vi "Decode Publish Package.vi"(8 "error in (no error)":errorcluster, 10 "PUBLISH in":refnum<class "PUBLISH.lvclass">, 11 "Server in":refnum<class "Server.lvclass">) -> (0 "error out":errorcluster, 1 "Payload":variant, 2 "Topic":string, 3 "Server out":refnum<class "Server.lvclass">)   [LabVIEW 2013, in "MQTT Server.lvlib" / "Server.lvclass"]
uses:
  Server.lvclass
  Control Packets/PUBLISH/PUBLISH.lvclass
  <vilib>/LabVIEW Open Source Project/Configuration Manager/Serializer/Serializer.lvclass
  Control Packets/ControlPacket/ControlPacket.lvclass/ControlPacket.ctl
  Control Packets/ControlPacket/ControlPacket.lvclass
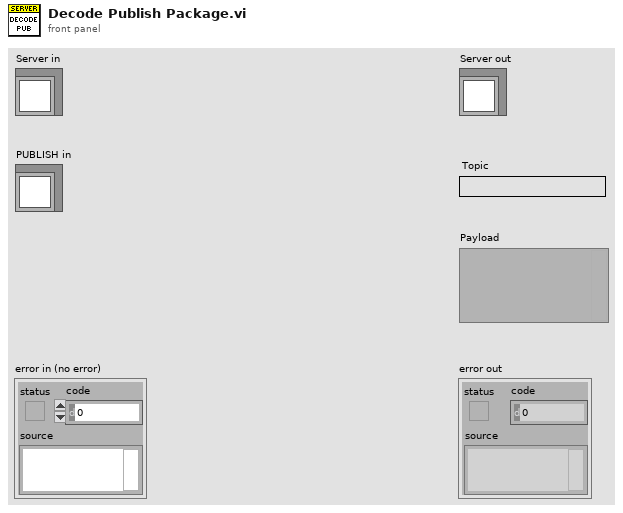
[diagram p1: front panel]
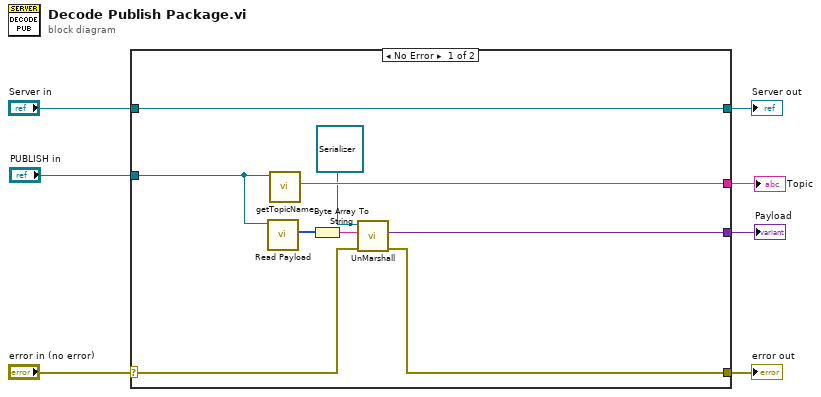
[diagram p0: block diagram]
diagram:
  n1 = case shown="No Error" "error in (no error)" {
    selector: "error in (no error)" -> [w9 w18]
    tunnel: [w8 w18] -> w6
    tunnel: [w16 w17] -> w4
    tunnel: "Server in" -> [w16 w17]
    tunnel: "PUBLISH in" -> [w14 _]
    tunnel: [w15 _] -> w2
    tunnel: [w10 _] -> w1
    frame No Error {
      n2 = call "Read Payload.vi"("ControlPacket in"=w14) -> ("Payload"=w13:u8[])  [unwired: 9 in, 1 out]
      n3 = call "getTopicName.vi"("PUBLISH in"=w14) -> ("Topic"=w15:string)  [unwired: 8 in, 2 out]
      n4 = Byte Array To String(unsigned byte array=w13) -> (string=w11:string)
      n5 = call-dynamic "UnMarshall.vi"("error in (no error)"=w9, "String"=w11, "Serializer in"=refnum<class "Serializer.lvclass"> refnum) -> ("error out"=w8:errorcluster, "Variant"=w10:variant)  [unwired: 6 in, 1 out]
    }
    frame Error {
    }
  }
  "error out" <- w6
  "Server out" <- w4
  "Topic" <- w2
  "Payload" <- w1
